vi "Timestamps_Init_CTR.vi"(8 "entrée d'erreur (pas d'erreur)":errorcluster) -> (0 "sortie d'erreur":errorcluster)   [LabVIEW 2026]
uses:
  <vilib>/DAQmx/create/channels.llb/DAQmx Create Channel (CI-Count Edges).vi
  <vilib>/DAQmx/configure/timing.llb/DAQmx Timing (Sample Clock).vi
  <resource>/objmgr/daqmx.rc
  controls/TypeDef_FGV.ctl
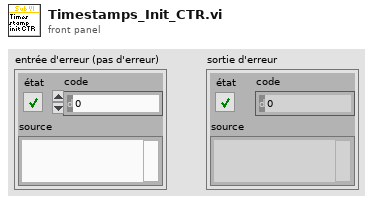
[diagram p1: front panel]
types:
  T1 = typedef "TypeDef_FGV.ctl" = enum16{"Initialize", "Add", "Read"}
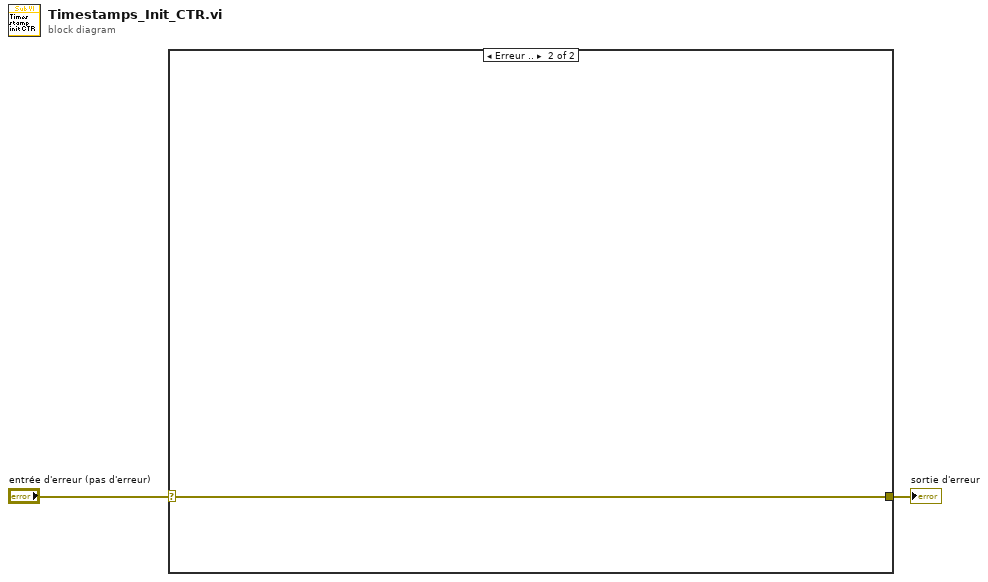
[diagram p0: block diagram]
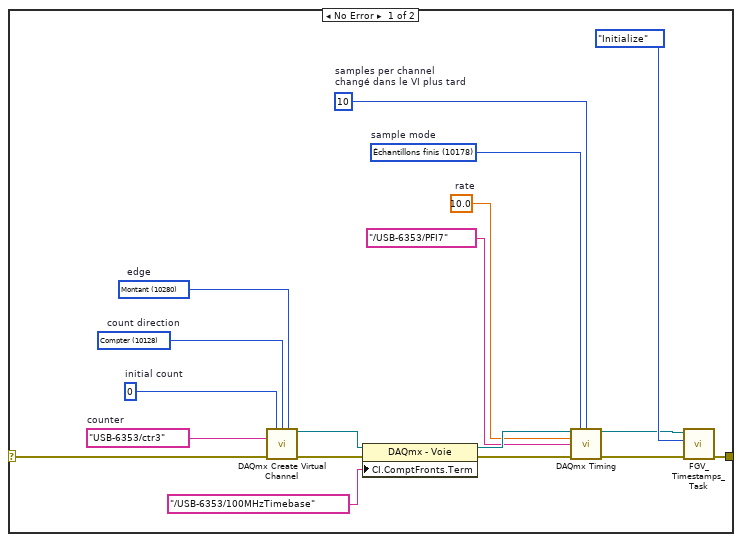
[diagram p2: hidden frame]
diagram:
  n1 = case shown="Erreur .." "entrée d'erreur (pas d'erreur)" {
    selector: "entrée d'erreur (pas d'erreur)" -> [w3 w21]
    tunnel: [w4 w21] -> w2
    frame No Error {
      w13 = 10  # samples per channel changé dans le VI plus tard
      w15 = 10.0  # rate
      w12 = 10178 items=["Échantillons finis"=10178, "Échantillons continus"=10123, "Point par point avec cadencement matériel"=12522]  # sample mode
      w11 = 10128 items=["Compter"=10128, "Compter à rebours"=10124, "Contrôlé de manière externe"=10326]  # count direction
      w10 = u32 0  # initial count
      w9 = 10280 items=["Montant"=10280, "Descendant"=10171]  # edge
      w8 = tag "USB-6353/ctr3"  # counter
      n2 = call-poly <vilib>:"DAQmx Create Virtual Channel.vi"("initial count"=w10, "count direction"=w11, "edge"=w9, "counter"=w8, "error in"=w3) -> ("task out"=w17:refnum<k21>, "error out"=w16:errorcluster)  [unwired: 9 in]
      n3 = property class="DAQmx - Voie"(reference=w17, error in=w16, "CI.ComptFronts.Term"=tag "/USB-6353/100MHzTimebase") -> (reference out=w18:refnum<k21>, error out=w19:errorcluster)
      n4 = call-poly <vilib>:"DAQmx Timing.vi"("task/channels in"=w18, "sample mode"=w12, "samples per channel"=w13, "rate"=w15, "source"=tag "/USB-6353/PFI7", "error in"=w19) -> ("task out"=w5:refnum<k21>, "error out"=w6:errorcluster)  [unwired: 8 in]
      n5 = call "FGV_Timestamps_Task.vi"("error in"=w6, "Action"=TypeDef_FGV."Initialize", "CTR Timestamps  task IN"=w5) -> ("error out"=w4:errorcluster)  [unwired: 7 in, 1 out]
    }
    frame Error {
    }
  }
  "sortie d'erreur" <- w2
